vi "Is Concrete Class.vi"(0 "SG Path Group in":refnum<class "SG Path Group.lvclass">, 11 "error in":errorcluster) -> (4 "SG Path Group out":refnum<class "SG Path Group.lvclass">, 6 "Is Concrete Class?":bool, 15 "error out":errorcluster)   [LabVIEW 2023, in "RFFixtureCharact.RMM.lvlib" / "SG Path Group.lvclass"]
uses:
  SG Path Group.lvclass
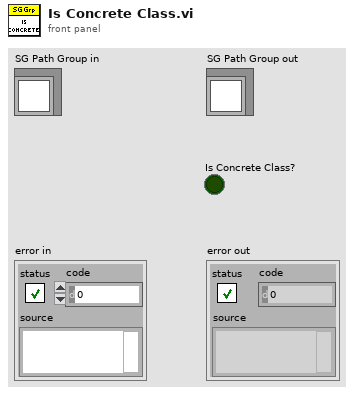
[diagram p1: front panel]
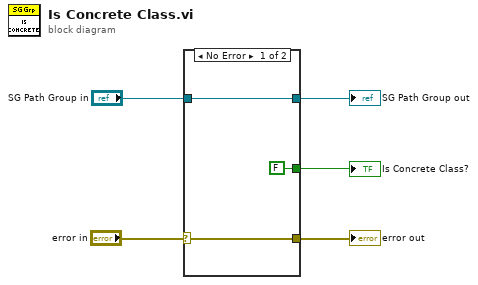
[diagram p0: block diagram]
diagram:
  n1 = case shown="No Error" "error in" {
    selector: "error in" -> [w7 w10]
    tunnel: [FALSE ("Is Concrete Class?") _] -> w3
    tunnel: [w7 w10] -> w5
    tunnel: [w6 w9] -> w2
    tunnel: "SG Path Group in" -> [w6 w9]
    frame No Error {
    }
    frame Error {
    }
  }
  "error out" <- w5
  "SG Path Group out" <- w2
  "Is Concrete Class?" <- w3
